vi "Test Base Does not Throw Error Using Hierarcical Separator in Name.vi"(8 "error in (no error)":errorcluster, 11 "Base Test in":refnum<class "Base Test.lvclass">) -> (0 "error out":errorcluster, 3 "Base Test out":refnum<class "Base Test.lvclass">)   [LabVIEW 2020, in "Base Test.lvclass"]
uses:
  Base Test.lvclass
  Base Test.lvclass/Base Test.ctl
  <vilib>/Astemes/LUnit/Test Case.lvclass
  Framework/Base/Base.lvclass
  C:/Program Files (x86)/National Instruments/LabVIEW 2020/vi.lib/Astemes/LUnit/Test Case.lvclass
  C:/Git/astemes-triarc-framework/source/Framework Test/Base Class Test/Base Test.lvclass
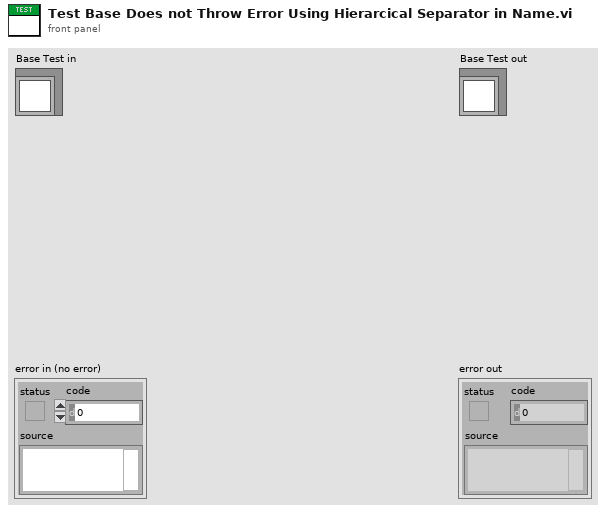
[diagram p1: front panel]
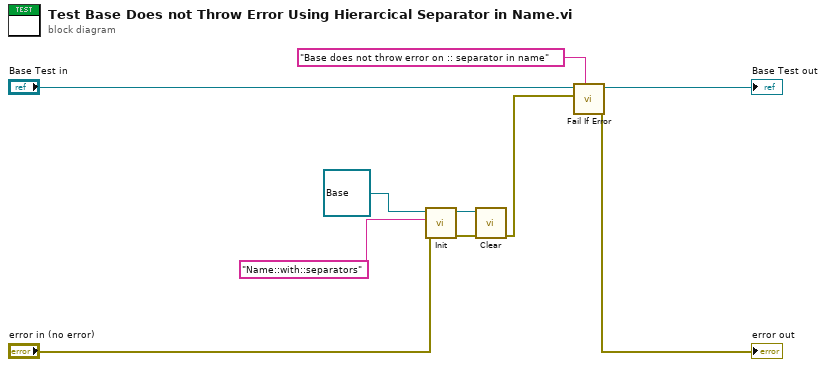
[diagram p0: block diagram]
diagram:
  n1 = call-dynamic "Init.vi"("error in (no error)"="error in (no error)", "Name"="Name::with::separators", "Base In"=refnum<class "Base.lvclass"> refnum) -> ("error out"=w6:errorcluster, "Base Out"=w2:refnum<class "Base.lvclass">)  [unwired: 7 in]
  n2 = call-dynamic "Clear.vi"("error in (no error)"=w6, "Base In"=w2) -> ("error out"=w3:errorcluster)  [unwired: 9 in]
  n3 = call <vilib>:"Fail If Error.vi"("Description"="Base does not throw error on :: separator in name", "Assert error"=w3, "LUnit Test Case In"="Base Test in") -> ("error out"=→"error out":errorcluster, "LUnit Test Case Out"=→"Base Test out":refnum<class "Base Test.lvclass">)  [unwired: 7 in]
